vi "Call Get HW Config.vi"(8 "error in":errorcluster, 10 "Refresh Modules":bool, 11 "serverName":string) -> (0 "error out":errorcluster, 3 "HW Config":T1)   [LabVIEW 2021, in "SEECD System Explorer.lvlib"]
uses:
  SEECD System Explorer.lvlib
  Type Defs/Host - HW Config.ctl
  Type Defs/Host - Local Chassis.ctl
  Type Defs/Host - Module.ctl
  Type Defs/IOV Container Contents.ctl
  Type Defs/Host - Master.ctl
  Type Defs/Host - Slave.ctl
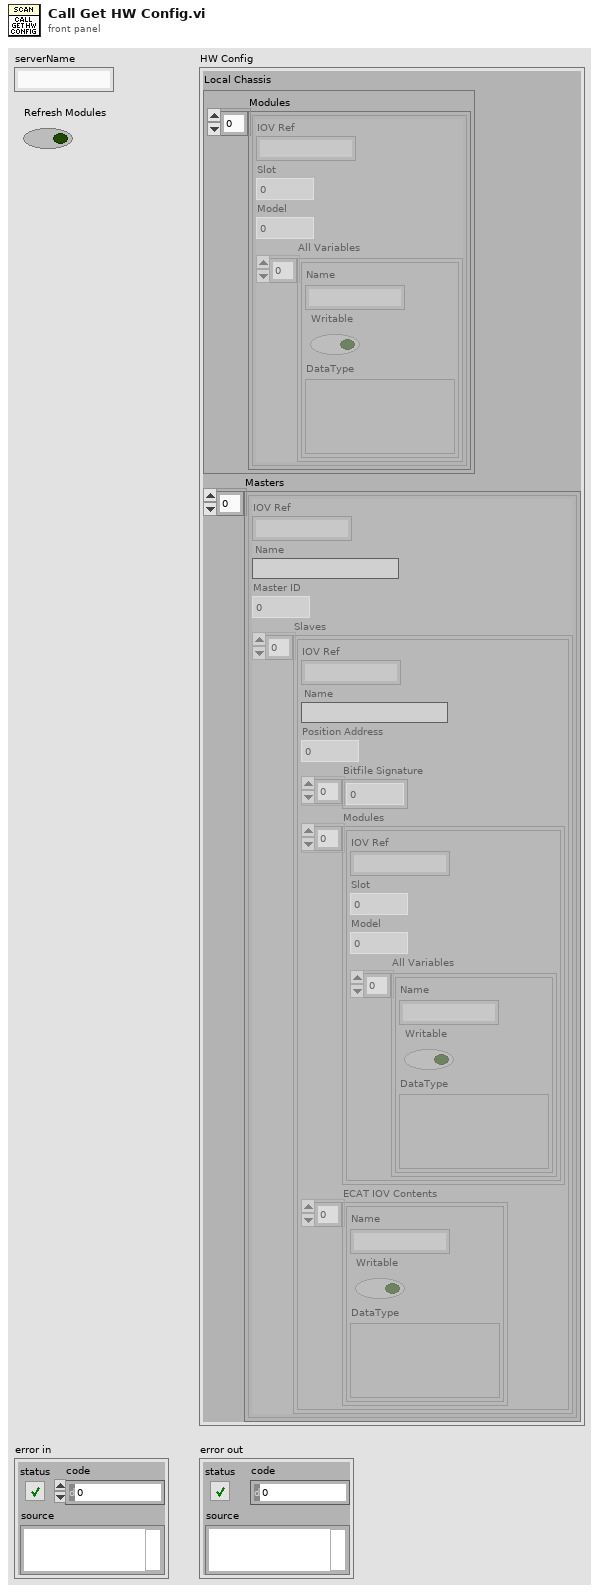
[diagram p1: front panel]
types:
  T1 = typedef "SEECD System Explorer.lvlib/Host - HW Config.ctl" = cluster{"Local Chassis":T2, "Masters":T5[]}
  T2 = typedef "SEECD System Explorer.lvlib/Host - Local Chassis.ctl" = cluster{"Modules":T3[]}
  T3 = typedef "SEECD System Explorer.lvlib/Host - Module.ctl" = cluster{"IOV Ref":string, "Slot":u32, "Model":u32, "All Variables":T4[]}
  T4 = typedef "SEECD System Explorer.lvlib/IOV Container Contents.ctl" = cluster{"Name":string, "Writable":bool, "DataType":variant}
  T5 = typedef "SEECD System Explorer.lvlib/Host - Master.ctl" = cluster{"IOV Ref":string, "Name":string, "Master ID":u32, "Slaves":T6[]}
  T6 = typedef "SEECD System Explorer.lvlib/Host - Slave.ctl" = cluster{"IOV Ref":string, "Name":string, "Position Address":u16, "Bitfile Signature":u8[], "Modules":T3[], "ECAT IOV Contents":T4[]}
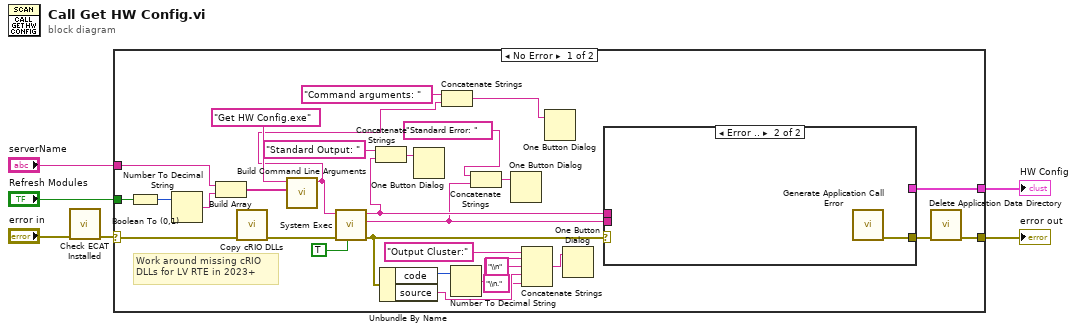
[diagram p0: block diagram]
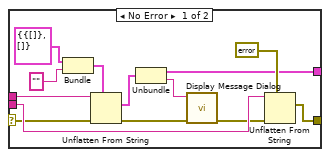
[diagram p2: hidden frame]
diagram:
  n1 = call "Check ECAT Installed.vi"("error in"="error in") -> ("error out"=w1:errorcluster)  [unwired: 10 in]
  n2 = case shown="No Error" w1 {
    selector: w1 -> [w35 w50]
    tunnel: [w24 w50] -> w6
    tunnel: "serverName" -> [w30 _]
    tunnel: [w34 _] -> w3
    tunnel: "Refresh Modules" -> [w28 _]
    frame No Error {
      # "Work around missing cRIO\nDLLs for LV RTE in 2023+"
      n3 = Boolean To (0,1)(Boolean=w28) -> (0, 1=w27:i16)
      n4 = Number To Decimal String(number=w27) -> (decimal integer string=w26:string)  [unwired: 1 in]
      n5 = Build Array(w30, w26) -> (w29:string[])
      n6 = call "Copy cRIO DLLs.vi"("error in"=w35) -> ("error out"=w25:errorcluster)  [unwired: 10 in]
      n7 = call "Build Command Line Arguments.vi"("Arguments"=w29, "Executable File Name"="Get HW Config.exe" ("name or relative path")) -> ("Command Line"=w8:string)  [unwired: 9 in]
      n8 = call <vilib>:"System Exec.vi"("run minimized? (F)"=TRUE, "error in (no error)"=w25, "command line"=w8) -> ("error out"=w17:errorcluster, "standard error"=w21:string, "standard output"=w22:string)  [unwired: 5 in, 1 out]
      n9 = Concatenate Strings("Standard Output: " ("string"), w22) -> (w19:string)
      n10 = Unbundle By Name(w17) -> ("code"=w14:i32, "source"=w11:string)
      n11 = One Button Dialog(message=w19) -> ()  [unwired: 1 in, 1 out]
      n12 = Concatenate Strings("Command arguments: " ("string"), w8) -> (w7:string)
      n13 = Number To Decimal String(number=w14) -> (decimal integer string=w13:string)  [unwired: 1 in]
      n14 = Concatenate Strings("Standard Error: " ("string"), w21) -> (w18:string)
      n15 = One Button Dialog(message=w18) -> ()  [unwired: 1 in, 1 out]
      n16 = Concatenate Strings("Output Cluster:" ("string"), w13, "\\n" ("string"), w11, "\\n." ("string")) -> (w16:string)
      n17 = One Button Dialog(message=w7) -> ()  [unwired: 1 in, 1 out]
      n18 = One Button Dialog(message=w16) -> ()  [unwired: 1 in, 1 out]
      n19 = case shown="Error .." w17 {
        selector: w17 -> [w45 _]
        tunnel: [w37 _] -> w34
        tunnel: [w47 w49] -> w33
        tunnel: w22 -> [w44 _]
        tunnel: w21 -> [w46 _]
        frame No Error {
          n20 = Bundle("HW Config"=T1 {"Local Chassis"={"Modules"=[]}, "Masters"=[]}, "") -> (w43:cluster{"HW Config":T1, string})  [unwired: 1 in]
          n21 = Unflatten From String(type=w43, binary string=w44, error in (no error)=w45) -> (value=w38:cluster{"HW Config":T1, string}, error out=w40:errorcluster)  [unwired: 2 in, 1 out]
          n22 = Unbundle(w38) -> ("HW Config"=w37:T1, w36:string)
          n23 = call "Display Message Dialog.vi"("error in"=w40, "Message to display"=w36) -> ("error out"=w39:errorcluster)  [unwired: 9 in]
          n24 = Unflatten From String(type=errorcluster {"status"=FALSE, "code"=0, "source"=""} ("error in (no error)"), binary string=w46, error in (no error)=w39) -> (value=w47:errorcluster)  [unwired: 2 in, 2 out]
        }
        frame Error {
          n25 = call "Generate Application Call Error.vi"() -> ("error out"=w49:errorcluster)  [unwired: 11 in]
        }
      }
      n26 = call "Delete Application Data Directory.vi"("error in"=w33) -> ("error out"=w24:errorcluster)  [unwired: 10 in]
    }
    frame Error {
    }
  }
  "HW Config" <- w3
  "error out" <- w6
